vi "The Plant and its parameters (WBDDO4).vi"() -> ()   [LabVIEW 2021]
uses:
  <vilib>/Utility/NIReport.llb/Report Type.ctl
  <vilib>/addons/control/pid/pid.llb/PID Advanced (DBL).vi
  <vilib>/Utility/file.llb/Write Delimited Spreadsheet (DBL).vi
  <vilib>/addons/control/pid/NI_PID_pid.lvlib
  <vilib>/Utility/NIReport.llb/NI_report.lvclass
  <vilib>/Utility/NIReport.llb/NI_ReportGenerationCore.lvlib
panel:
  in  "Plant Parameters":T1={"Static Gain"=2.5, "lag (s)"=4.0, "deadtime (s)"=0.1, "load"=40.0, "deadband"=2.0, "sensor noise"=0.25, "initial PV"=0.0, "plant noise"=1.0}
  out "Waveform Chart 2":dbl[](graph)
  out "U-1":dbl
  out "U":dbl
  in  "stop":bool
  out "output array":dbl[][](array[numeric])
  out "Error test":bool
  out "Waveform Chart":T2(graph)
  out "Valve":bool
  in  "PID parameters":cluster{" K":dbl, "Ti min":dbl, "Td, min":dbl}={" K"=3.5, "Ti min"=0.005, "Td, min"=0.0} {"Td, min" format="%.3f"; "Ti min" format="%.3f"; "K" format="%.3f"}
  out "Tank level":dbl format="%.2f"
  in  "Plant dt (s)":dbl=1.0 format="%.3f"
  in  "Setpoint":dbl=20.0 format="%.2f"
  in  "Integrator ? 2":bool
  in  "reinitialize? (F) 2":bool
  out "Tank level":dbl(slide) scale=0.0..100.0
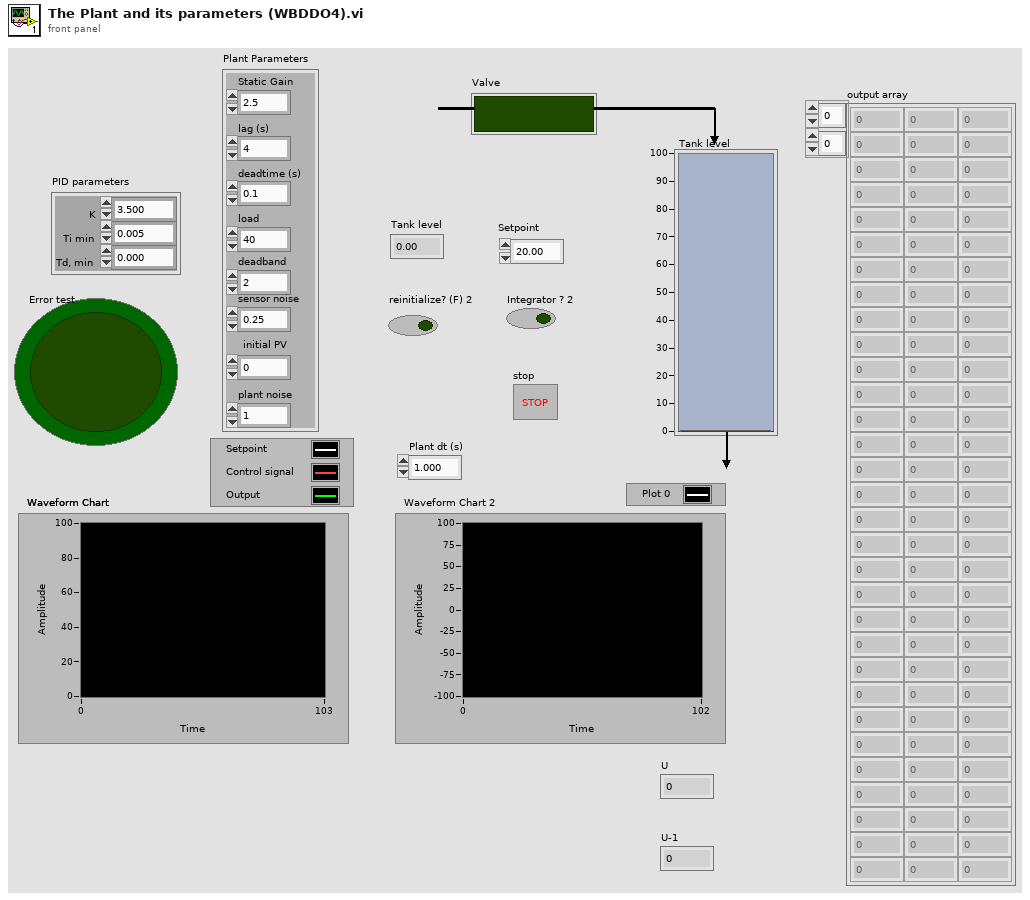
[diagram p1: front panel]
types:
  T1 = cluster{"Static Gain":dbl, "lag (s)":dbl, "deadtime (s)":dbl, "load":dbl, "deadband":dbl, "sensor noise":dbl, "initial PV":dbl, "plant noise":dbl}
  T2 = cluster{"Setpoint":dbl, "output":dbl, "Plant Output":dbl}
  T3 = typedef "NI_ReportGenerationCore.lvlib/Report Type.ctl" = enum16{"HTML", "Word", "Excel"}
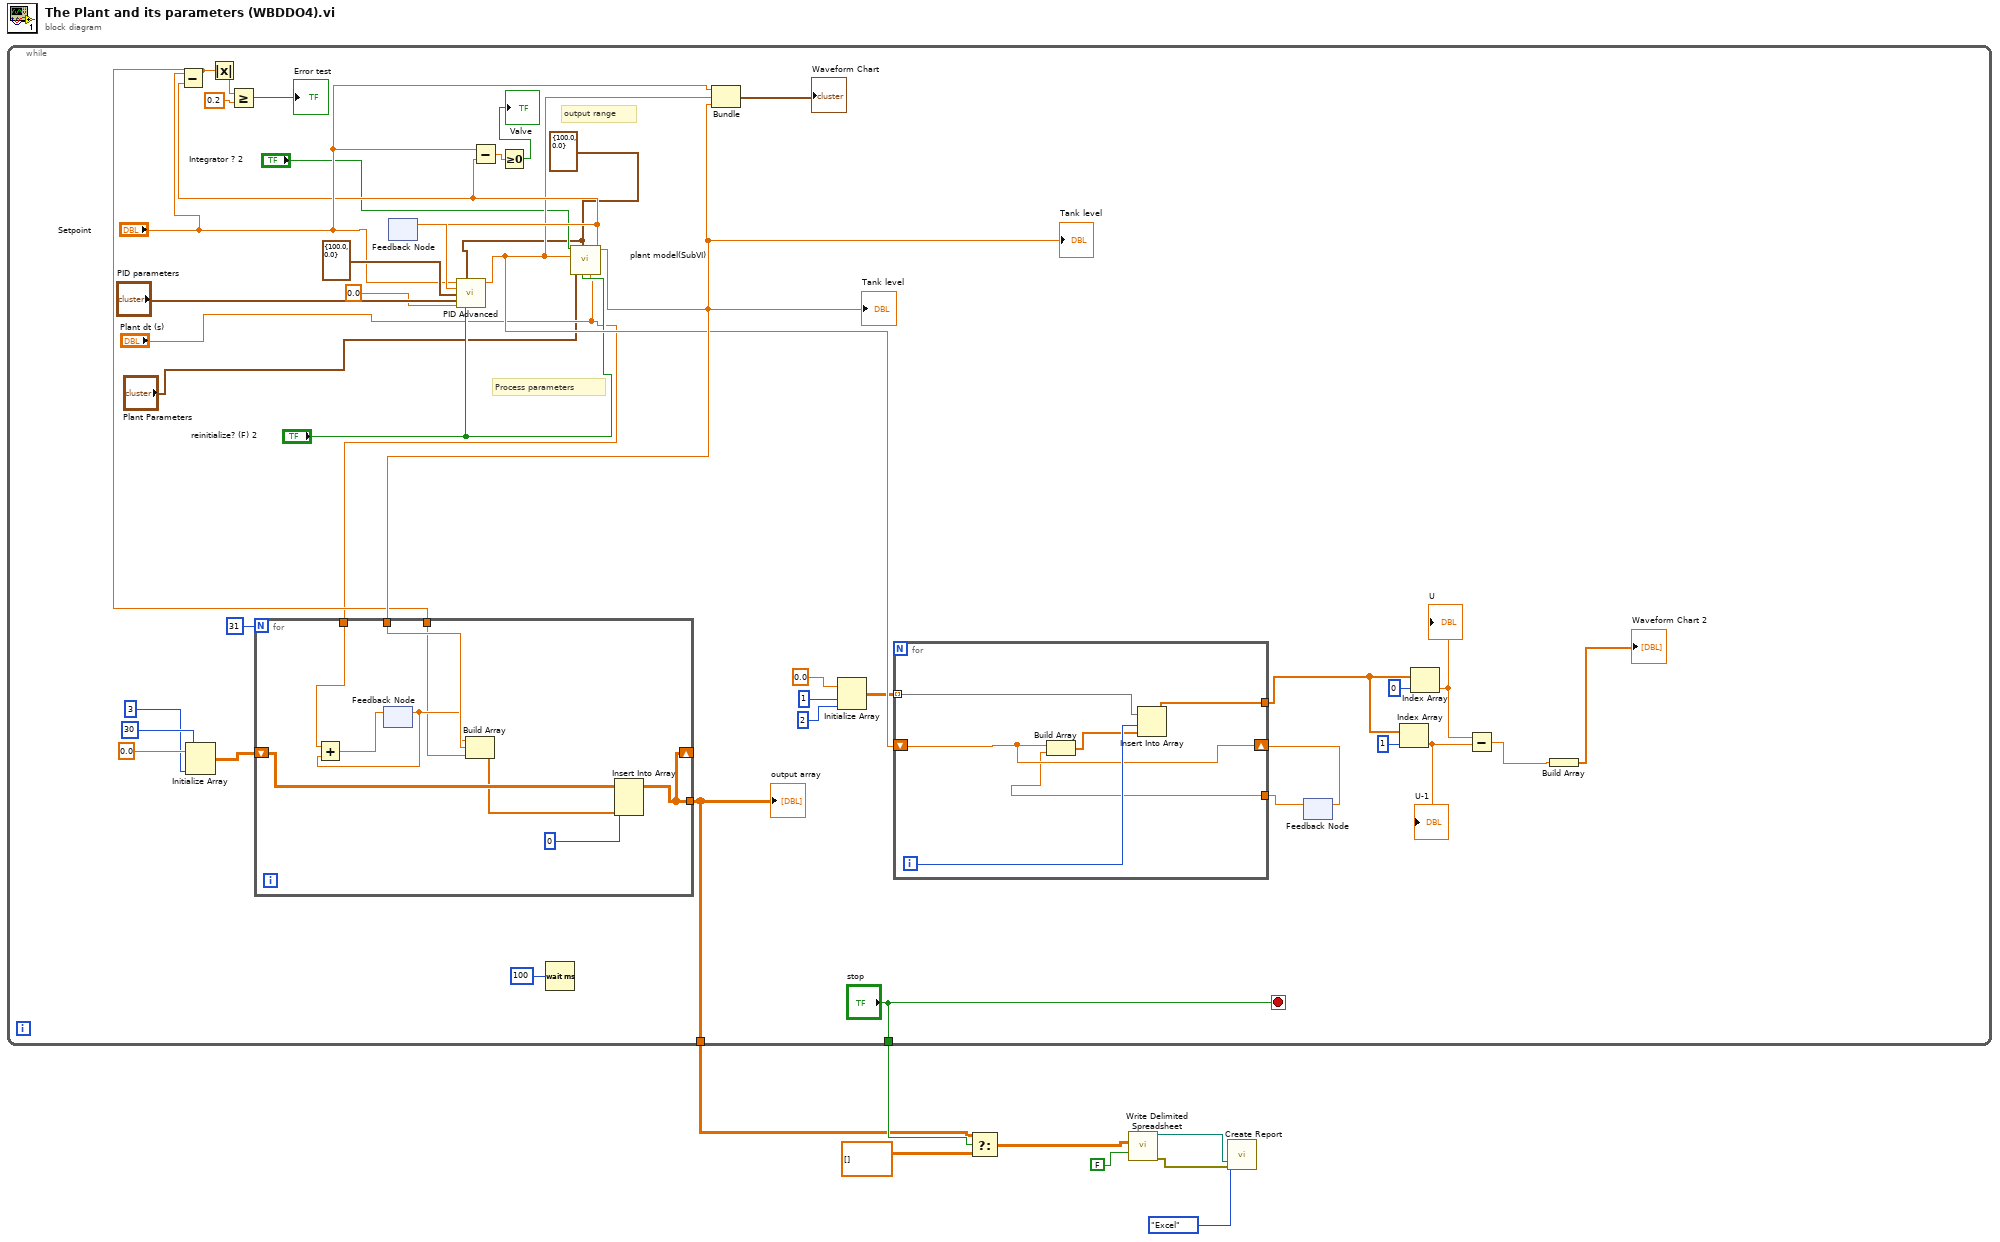
[diagram p0: block diagram]
diagram:
  n1 = while {
    tunnel: ["stop"] -> w8
    tunnel: [w14] -> w7
    stop <- "stop" stop-if-true
    w10 = cluster{"output high":dbl, "output low":dbl} {"output high"=100.0, "output low"=0.0} ("output saturation range")
    # "Process parameters"
    # "output range"
    n2 = Initialize Array(0.0 ("element"), 30 ("dimension size"), 3 ("dimension size")) -> (w38:dbl[][])
    n3 = feedback #1() -> (w48:dbl)  [unwired: 1 in]
    n4 = call-poly <vilib>:"PID Advanced.vi"("setpoint"="Setpoint", "output range"=w10, "process variable"=w48, "setpoint range"=cluster{"setpoint high":dbl, "setpoint low":dbl} {"setpoint high"=100.0, "setpoint low"=0.0}, "PID gains"="PID parameters", "dt (s)"=0.0, "reinitialize? (F)"="reinitialize? (F) 2") -> ("output"=w30:dbl)  [unwired: 7 in, 1 out]
    n5 = Wait (ms)(milliseconds to wait=u32 100) -> ()  [unwired: 1 out]
    n6 = call "plant model(SubVI).vi"("dt (s)"="Plant dt (s)", "reinitialize? (F)"="reinitialize? (F) 2", "output saturation range"=w10, "process parameters"="Plant Parameters", "Plant Input"=w30, "Integrator ?"="Integrator ? 2") -> ("Plant Output"=w33:dbl)  [unwired: 5 in]
    "Tank level" <- w33
    "Tank level" <- w33
    n7 = Subtract(x="Setpoint", y=w33) -> (x-y=w32:dbl)
    n8 = Absolute Value(x=w32) -> (abs(x)=w41:dbl)
    n9 = Greater Or Equal?(x=w41, y=0.2) -> (x >= y?=→"Error test":bool)
    n10 = for {
      N: 31 -> [_]
      shift-right: [w55] -> _
      shift-left: w38 -> [w62]
      tunnel: w33 -> [w63]
      tunnel: "Plant dt (s)" -> [w60]
      tunnel: [w55] -> w14
      tunnel: w32 -> [w56]
      n11 = feedback #2() -> (w58:dbl)  [unwired: 1 in]
      n12 = Add(x=w60, y=w58) -> (x+y=w59:dbl)
      n13 = feedback-in #2(w59) -> ()
      n14 = Build Array(w58, w63, w56) -> (w61:dbl[])
      n15 = Insert Into Array(array=w62, index (row)=0, new element=w61) -> (w55:dbl[][])  [unwired: 1 in]
    }
    "output array" <- w14
    n16 = feedback-in #1(w33) -> ()
    n17 = Subtract(x="Setpoint", y=w33) -> (x-y=w45:dbl)
    n18 = Greater Or Equal To 0?(x=w45) -> (x >= 0?=→"Valve":bool)
    n19 = Bundle("Setpoint"="Setpoint", "output"=w30, "Plant Output"=w33) -> (→"Waveform Chart":T2)  [unwired: 1 in]
    n20 = Initialize Array(0.0 ("element"), 1 ("dimension size"), 2 ("dimension size")) -> (w26:dbl[][])
    n21 = feedback #3() -> (w25:dbl)  [unwired: 1 in]
    n22 = for {
      shift-right: [w51] -> w24
      shift-left: w30 -> [w51]
      tunnel: w26 -> [w52] mode=indexing
      tunnel: [w50] -> w20
      tunnel: w25 -> [w49]
      i -> [w54]
      n23 = Build Array(w51, w49) -> (w53:dbl[])
      n24 = Insert Into Array(array=w52, index=w54, new element=w53) -> (w50:dbl[])
    }
    n25 = feedback-in #3(w24) -> ()
    n26 = Index Array(array=w20, index=1) -> (element=w21:dbl)
    "U-1" <- w21
    n27 = Index Array(array=w20, index=0) -> (element=w19:dbl)
    "U" <- w19
    n28 = Subtract(x=w19, y=w21) -> (x-y=w18:dbl)
    n29 = Build Array(w18) -> (→"Waveform Chart 2":dbl[])
  }
  n30 = Select(t=w7, s=w8, f=dbl[][] []) -> (s? t:f=w6:dbl[][])
  n31 = call-poly <vilib>:"Write Delimited Spreadsheet.vi"("2D data"=w6, "append to file? (new file:F)"=FALSE) -> ("new file path (Not A Path if cancelled)"=w1:path, "error out"=w2:errorcluster)  [unwired: 12 in]
  n32 = call <vilib>:"Create Report.vi"("report type"=Report_Type."Excel", "template (empty)"=w1, "error in (no error)"=w2) -> ()  [unwired: 11 in, 2 out]
